vi "CSDBTools.Main.vi"() -> ()   [LabVIEW 2014]
doc: "Starter VI for the CS database and tag tools.\n\nPlease note, that this tool must not run together with CS in the same LabVIEW execution system.\n\nLicense Agreement for this software:\n\nCopyright (C)\nGesellschaft für Schwerionenforschung, GSI\nPlanckstr. 1\n64291 Darmstadt\nGermany\n\nContact: D.Beck@gsi.de \n\nThis program is free software; you can redistribute it and/or modify it under the terms of the \nGNU General Public License as published by the Free Software Foundation; either version 2 of \nthe license, or (at your option) any later version.\n\nThis program is distributed in the hope that it will be useful, but WITHOUT ANY WARRANTY; \nwithout even the implied warranty of MERCHANTABILITY or FITNESS FOR A PARTICULAR PURPOSE. See the GNU General License for more details (http://www.gnu.org).\n\nGesellschaft für Schwerionenforschung, GSI\nPlanckstr. 1, 64291 Darmstadt, Germany\nFor all questions and ideas contact: M.Richter@gsi.de, H.Brand@gsi.de or D.Beck@gsi.de.\nLast update: 16-JUN-2004"
uses:
  CSDB_Transfer/CSDB_Transfer.lvlib
  CSDB_Config/CSDB_Config.lvlib
  CSDB_SVEdit/CSDB_SVEdit.lvlib
  CSDB_Common/CSDB_Common.lvlib
panel:
  out "nameAndVersion":string
  in  "SVEditor":bool
  in  "Convert DB":bool
  in  "Database and Tag Tools":bool
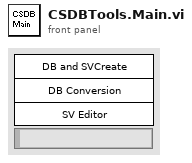
[diagram p1: front panel]
types:
  T1 = enum32{"invalid app kind", "Development System", "Run Time System", "Student Edition", "Embedded LabVIEW", "Evaluation", "Custom"}
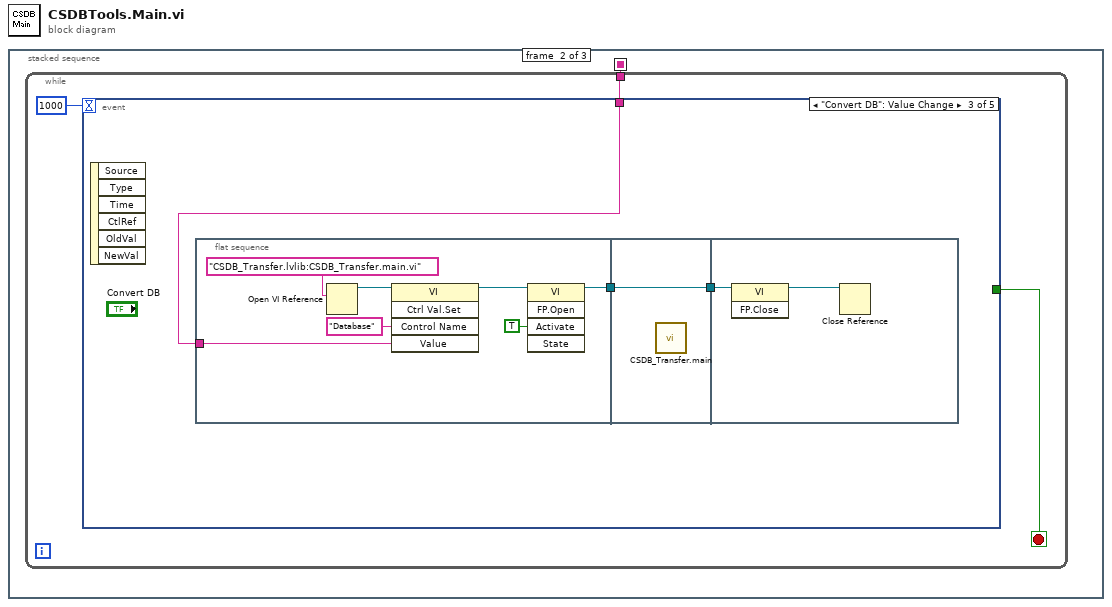
[diagram p0: block diagram]
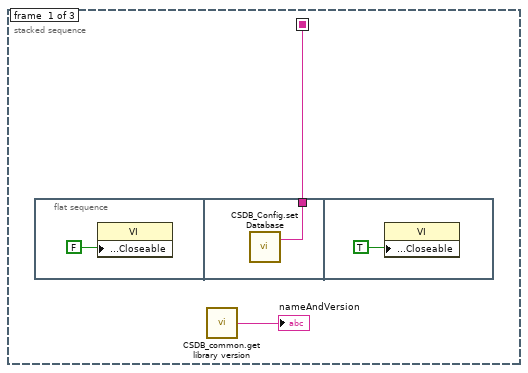
[diagram p2: hidden frame]
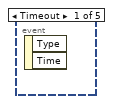
[diagram p3: hidden frame]
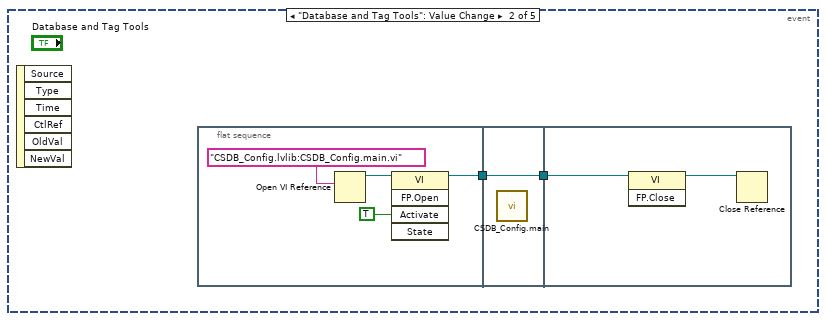
[diagram p4: hidden frame]
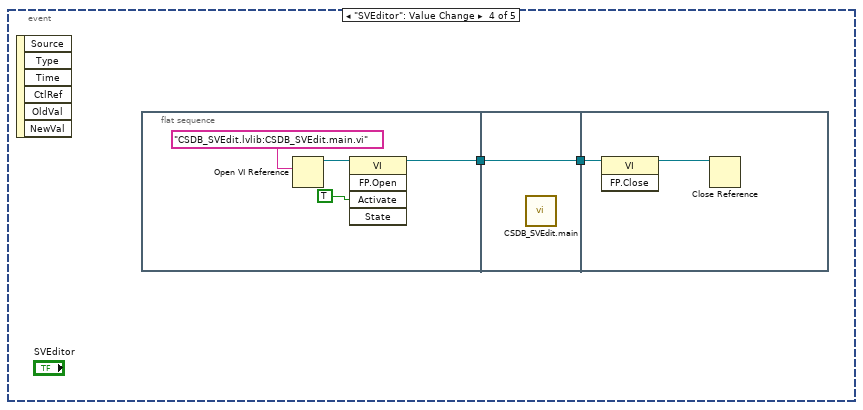
[diagram p5: hidden frame]
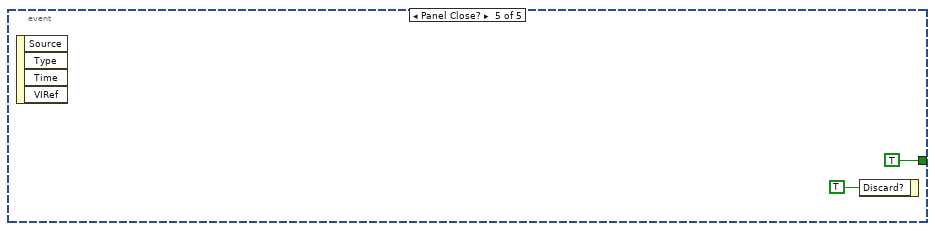
[diagram p6: hidden frame]
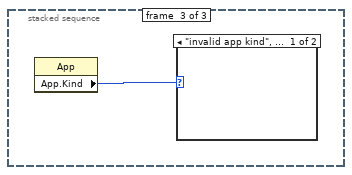
[diagram p7: hidden frame]
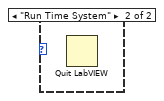
[diagram p8: hidden frame]
diagram:
  n1 = stacked-sequence {
    seq-local: [w1 _ _] -> [_ w6 _]
    frame #0 {
      n2 = flat-sequence {
        tunnel: [w4] -> w1
        frame #0 {
          n3 = property class="VI"("Front Panel.Closeable"=FALSE ("Front Panel Window:Closeable")) -> ()  [unwired: 2 in, 2 out]
        }
        frame #1 {
          n4 = call "CSDB_Config.set Database.vi"() -> ("Database"=w4:string)  [unwired: 18 in, 1 out]
        }
        frame #2 {
          n5 = property class="VI"("Front Panel.Closeable"=TRUE ("Front Panel Window:Closeable")) -> ()  [unwired: 2 in, 2 out]
        }
      }
      n6 = call "CSDB_common.get library version.vi"() -> ("nameAndVersion"=→"nameAndVersion":string)  [unwired: 1 in]
    }
    frame #1 {
      n7 = while {
        tunnel: w6 -> [w7]
        stop <- w9 stop-if-true
        n8 = event shown="[2] \"Convert DB\": Value Change" {
          selector: _ -> [_ _ _ _ _]
          dyn-events: _ -> [_ _ _ _ _]
          timeout: 1000 -> [_ _ _ _ _]
          tunnel: [_ _ _ _ TRUE ("Stop")] -> w9
          tunnel: w7 -> [_ _ w19 _ _]
          event Timeout {
            n9 = event-data() -> ()  [unwired: 1 in, 2 out]
          }
          event "Database and Tag Tools": Value Change {
            n10 = event-data() -> ()  [unwired: 1 in, 6 out]
            n11 = flat-sequence {
              tunnel: [w14] -> w10
              tunnel: [w16] -> w11
              tunnel: w10 -> [w16]
              tunnel: w11 -> [w18]
              frame #0 {
                n12 = Open VI Reference(vi path="CSDB_Config.lvlib:CSDB_Config.main.vi") -> (vi reference=w15:refnum<vi>)  [unwired: 5 in, 1 out]
                n13 = invoke class="VI" method="FP.Open"(reference=w15, "Activate"=TRUE) -> (reference out=w14:refnum<vi>)  [unwired: 3 in, 4 out]
              }
              frame #1 {
                n14 = call "CSDB_Config.main.vi"() -> ()  [unwired: 20 in]
              }
              frame #2 {
                n15 = invoke class="VI" method="FP.Close"(reference=w18) -> (reference out=w17:refnum<vi>)  [unwired: 2 in, 2 out]
                n16 = Close Reference(reference=w17) -> ()  [unwired: 1 in, 1 out]
              }
            }
          }
          event "Convert DB": Value Change {
            n17 = event-data() -> ()  [unwired: 1 in, 6 out]
            n18 = flat-sequence {
              tunnel: [w28] -> w20
              tunnel: w19 -> [w22]
              tunnel: [w29] -> w21
              tunnel: w20 -> [w29]
              tunnel: w21 -> [w31]
              frame #0 {
                n19 = Open VI Reference(vi path="CSDB_Transfer.lvlib:CSDB_Transfer.main.vi") -> (vi reference=w25:refnum<vi>)  [unwired: 5 in, 1 out]
                n20 = invoke class="VI" method="Ctrl Val.Set"(reference=w25, "Control Name"="Database", "Value"=w22) -> (reference out=w24:refnum<vi>)  [unwired: 2 in, 4 out]
                n21 = invoke class="VI" method="FP.Open"(reference=w24, "Activate"=TRUE) -> (reference out=w28:refnum<vi>)  [unwired: 3 in, 4 out]
              }
              frame #1 {
                n22 = call "CSDB_Transfer.main.vi"() -> ()  [unwired: 20 in]
              }
              frame #2 {
                n23 = invoke class="VI" method="FP.Close"(reference=w31) -> (reference out=w30:refnum<vi>)  [unwired: 2 in, 2 out]
                n24 = Close Reference(reference=w30) -> ()  [unwired: 1 in, 1 out]
              }
            }
          }
          event "SVEditor": Value Change {
            n25 = event-data() -> ()  [unwired: 1 in, 6 out]
            n26 = flat-sequence {
              tunnel: [w36] -> w32
              tunnel: [w38] -> w33
              tunnel: w32 -> [w38]
              tunnel: w33 -> [w40]
              frame #0 {
                n27 = Open VI Reference(vi path="CSDB_SVEdit.lvlib:CSDB_SVEdit.main.vi") -> (vi reference=w37:refnum<vi>)  [unwired: 5 in, 1 out]
                n28 = invoke class="VI" method="FP.Open"(reference=w37, "Activate"=TRUE) -> (reference out=w36:refnum<vi>)  [unwired: 3 in, 4 out]
              }
              frame #1 {
                n29 = call "CSDB_SVEdit.main.vi"() -> ()  [unwired: 1 in]
              }
              frame #2 {
                n30 = invoke class="VI" method="FP.Close"(reference=w40) -> (reference out=w39:refnum<vi>)  [unwired: 2 in, 2 out]
                n31 = Close Reference(reference=w39) -> ()  [unwired: 1 in, 1 out]
              }
            }
          }
          event Panel Close? {
            n32 = event-data() -> ()  [unwired: 1 in, 4 out]
            n33 = event-data("Discard?"=TRUE) -> ()  [unwired: 1 in, 1 out]
          }
        }
      }
    }
    frame #2 {
      n34 = property class="App"() -> ("App.Kind"=w43:T1)  [unwired: 2 in, 2 out]
      n35 = case shown="\"invalid app kind\", Default" w43 {
        frame "invalid app kind", Default {
        }
        frame "Run Time System" {
          n36 = Quit LabVIEW() -> ()  [unwired: 1 in]
        }
      }
    }
  }
